vi "Shutdown.vi"(6 "timeout in ms (3000)":i32=3000, 7 "Wait for reponse (F)":bool, 8 "error in (no error)":errorcluster, 11 "Parallel Process in":refnum<class "Parallel Process.lvclass">) -> (0 "error out":errorcluster, 3 "Parallel Process out":refnum<class "Parallel Process.lvclass">)   [LabVIEW 2011, in "Messenging.lvlib" / "Parallel Process.lvclass"]
uses:
  Parallel Process.lvclass
  Interprocess Messenger/Send/Send.lvclass
  Interprocess Messenger/TextVarientMessage/MSG.lvclass
  Interprocess Messenger/TextVarientMessage/Write (no data).vi
  Interprocess Messenger/Send/Send Message.vi
  Interprocess Messenger/Send/Query (static).vi
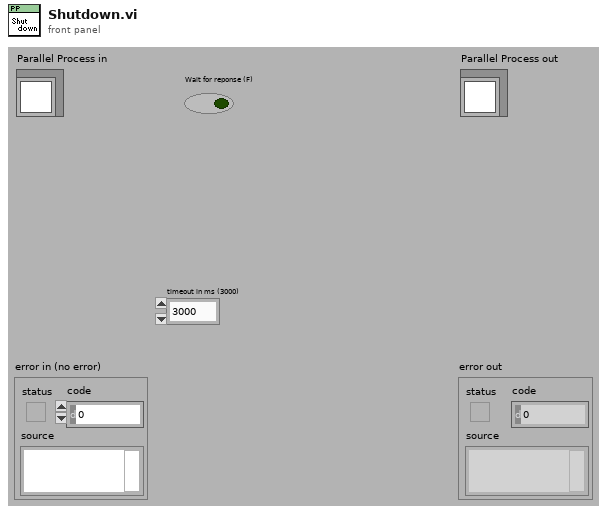
[diagram p1: front panel]
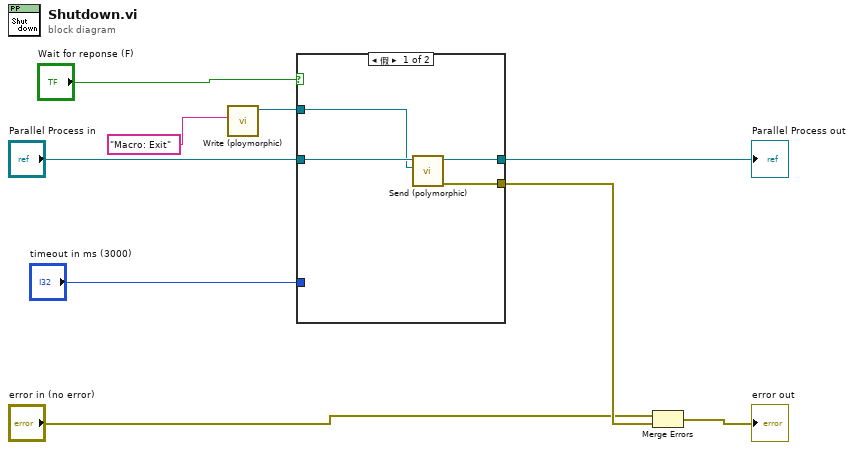
[diagram p0: block diagram]
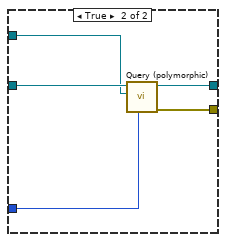
[diagram p2: hidden frame]
diagram:
  n1 = call-poly "Write (ploymorphic).vi"("Label"="Macro: Exit" ("Command String")) -> ("Message"=w4:refnum<class "MSG.lvclass">)  [unwired: 1 in, 9 out]
  n2 = case shown="假" "Wait for reponse (F)" {
    tunnel: [w11 w16] -> w9
    tunnel: [w12 w17] -> w8
    tunnel: "timeout in ms (3000)" -> [_ w14]
    tunnel: "Parallel Process in" -> [w13 w18]
    tunnel: w4 -> [w10 w15]
    frame False {
      n3 = call-poly "Send (polymorphic).vi"("Message"=w10, "MSR Parent in"=w13) -> ("error out"=w11:errorcluster, "MSR Parent out"=w12:refnum<class "Parallel Process.lvclass">)  [unwired: 1 in, 7 out]
    }
    frame True {
      n4 = call-poly "Query (polymorphic).vi"("timeout in ms (5000)"=w14, "Message"=w15, "MSR Parent"=w18) -> ("error out"=w16:errorcluster, "MSR Parent"=w17:refnum<class "Parallel Process.lvclass">)  [unwired: 3 in, 4 out]
    }
  }
  "Parallel Process out" <- w8
  n5 = Merge Errors("error in (no error)", w9) -> (→"error out":errorcluster)
